vi "Read Channel.vi"(8 "error in (no error)":errorcluster, 11 "PSU in":refnum<class "PSU.lvclass">) -> (0 "error out":errorcluster, 2 "Channel":string, 3 "PSU out":refnum<class "PSU.lvclass">)   [LabVIEW 2014, in "PSU.lvclass"]
uses:
  PSU.lvclass
  PSU.lvclass/PSU.ctl
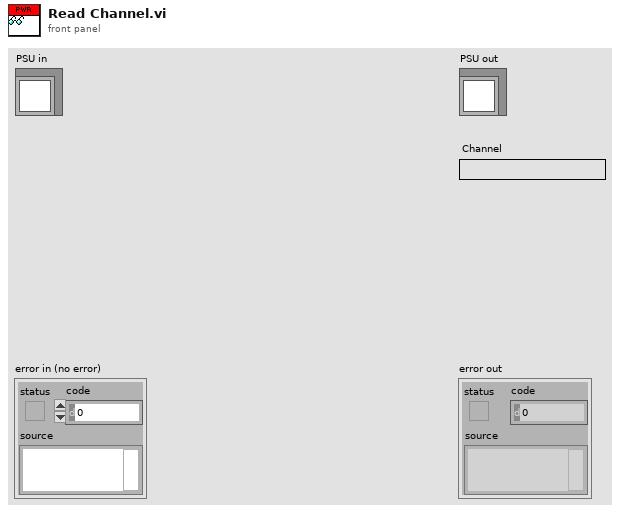
[diagram p1: front panel]
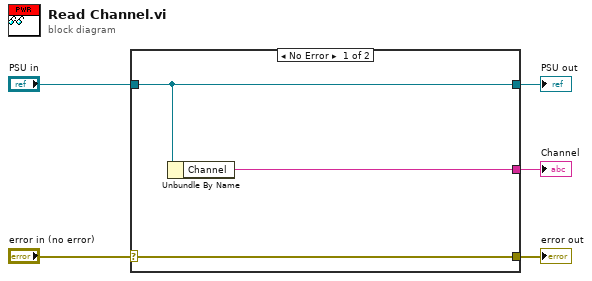
[diagram p0: block diagram]
diagram:
  n1 = case shown="No Error" "error in (no error)" {
    selector: "error in (no error)" -> [w8 w9]
    tunnel: [w8 w9] -> w4
    tunnel: [w7 w10] -> w2
    tunnel: "PSU in" -> [w7 w10]
    tunnel: [w6 _] -> w1
    frame No Error {
      n2 = Unbundle By Name(w7) -> ("Channel"=w6:string)
    }
    frame Error {
    }
  }
  "error out" <- w4
  "PSU out" <- w2
  "Channel" <- w1
